vi "DSF.Engine.Sequencer.Set Plugin Bundles.vi"(8 "error in (no error)":errorcluster, 10 "Plugin Bundles":refnum<class "DSF.Engine.Sequencer.Timing Bundle.lvclass">[](array[class]), 11 "Sequencer in":refnum<class "DSF.Engine.Sequencer.lvclass">) -> (0 "error out":errorcluster, 3 "Sequencer out":refnum<class "DSF.Engine.Sequencer.lvclass">)   [LabVIEW 2017, in "DSF.Engine.lvlib" / "DSF.Engine.Sequencer.lvclass"]
uses:
  DSF.Engine.Sequencer.lvclass
  DSF.Engine.Sequencer.Timing Bundle.lvclass
  DSF.Engine.Sequencer.lvclass/DSF.Engine.Sequencer.ctl
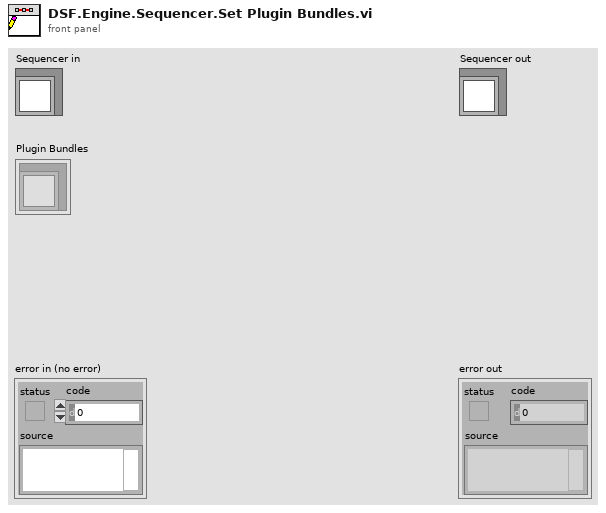
[diagram p1: front panel]
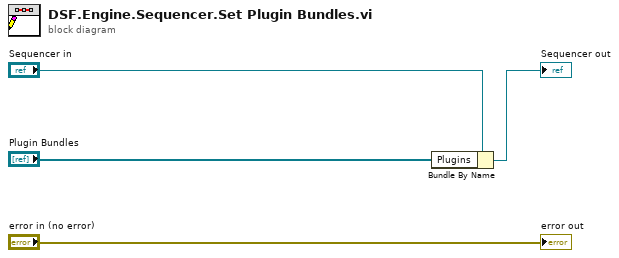
[diagram p0: block diagram]
diagram:
  n1 = Bundle By Name(cluster="Sequencer in", "Plugins"="Plugin Bundles") -> (→"Sequencer out":refnum<class "DSF.Engine.Sequencer.lvclass">)
  "error out" <- "error in (no error)"
